vi "display permission to classification.vi"(11 "display permissions":T1) -> (3 "channel classification":T2)   [LabVIEW 2013, in "Shared Library Module editor node.lvclass"]
doc: "Platypus Framework 1.0.1.60\nNI Systems Engineering - National Instruments"
uses:
  Shared Library Module editor node.lvclass
  <vilib>/NI/Tag Bus Module Framework/channel/channel classification.ctl
  permissions.ctl
  <vilib>/NI/Tag Bus Module Framework/channel/TBM channel.lvclass
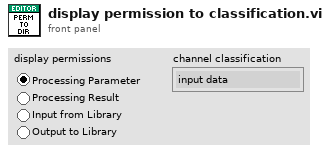
[diagram p1: front panel]
types:
  T1 = typedef "Shared Library Module editor node.lvclass/permissions.ctl" = enum32{"Processing Parameter", "Processing Result", "Input from Library", "Output to Library"}
  T2 = typedef "TBM channel.lvclass/channel classification.ctl" = enum16{"input data", "output data", "processing parameter", "processing result"}
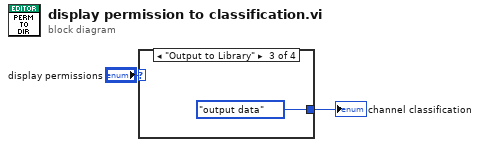
[diagram p0: block diagram]
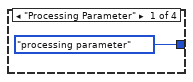
[diagram p2: hidden frame]
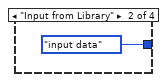
[diagram p3: hidden frame]
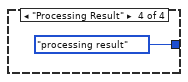
[diagram p4: hidden frame]
diagram:
  n1 = case shown="\"Output to Library\"" "display permissions" {
    tunnel: [channel_classification."processing parameter" ("channel classification") channel_classification."input data" ("channel classification") channel_classification."output data" ("channel classification") channel_classification."processing result" ("channel classification")] -> w2
    frame "Processing Parameter" {
    }
    frame "Input from Library" {
    }
    frame "Output to Library" {
    }
    frame "Processing Result" {
    }
  }
  "channel classification" <- w2
